vi "do_on_loop.vi"(1 "loopsToSkip":dbl, 2 "loopIteration":dbl) -> (0 "x = 0?":bool)   [LabVIEW 2012]
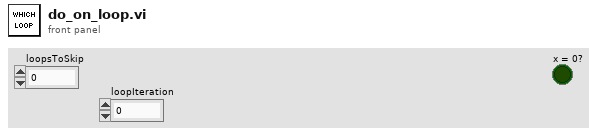
[diagram p1: front panel]
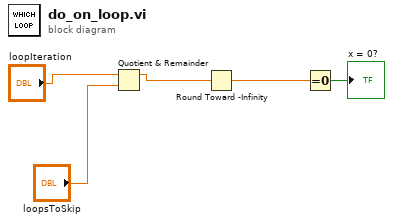
[diagram p0: block diagram]
diagram:
  n1 = Quotient & Remainder(x="loopIteration", y="loopsToSkip") -> (x-y*floor(x/y)=w3:dbl)  [unwired: 1 out]
  n2 = Round Toward -Infinity(1:w3) -> (0:w2:dbl)
  n3 = Equal To 0?(x=w2) -> (x = 0?=→"x = 0?":bool)
